vi "Conditional String Reverse.vi"(7 "Search Start Point":T1, 11 "String in":string) -> (3 "String out":string)   [LabVIEW 2017, in "SSH.lvlib"]
doc: "Reverses the string if the start point is set to the end"
uses:
  SSH.lvlib
  Search Start Point.ctl
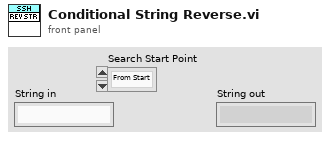
[diagram p1: front panel]
types:
  T1 = typedef "SSH.lvlib/Search Start Point.ctl" = enum16{"From Start", "From End"}
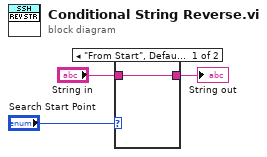
[diagram p0: block diagram]
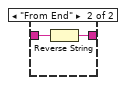
[diagram p2: hidden frame]
diagram:
  n1 = case shown="\"From Start\", Default" "Search Start Point" {
    tunnel: "String in" -> [w4 w6]
    tunnel: [w4 w5] -> w2
    frame "From Start", Default {
    }
    frame "From End" {
      n2 = Reverse String(1:w6) -> (0:w5:string)
    }
  }
  "String out" <- w2
